vi "Optical Flow Example.vi"() -> ()   [LabVIEW 2011]
uses:
  <vilib>/vision/NI_Vision_Development_Module.lvlib
panel:
  out "Image":T1(plugin-control)
  in  "stop":bool
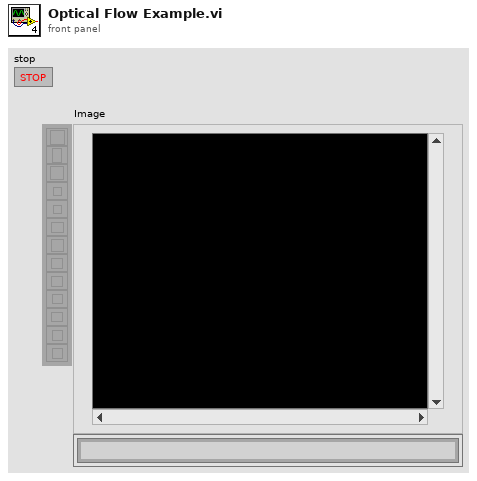
[diagram p1: front panel]
types:
  T1 = typedef "IMAQ Image.ctl" = refnum<image>
  T2 = typedef "Image Type" = u32
  T3 = typedef "t_CallbackReferences.ctl" = cluster{"LV event callback ":refnum<k27>, "Proxy instance":refnum<k24>, "(*f)(...)":i32}
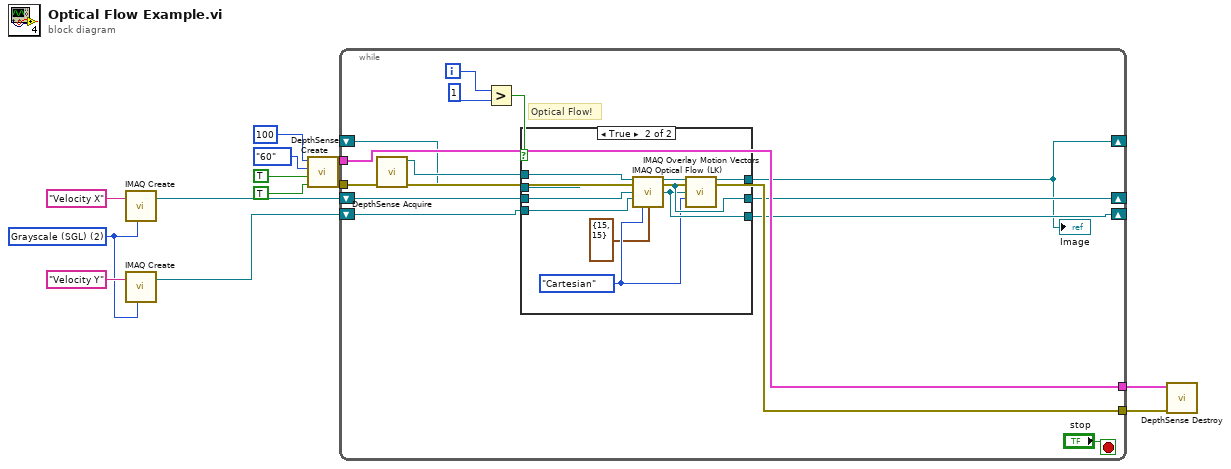
[diagram p0: block diagram]
diagram:
  w3 = T2 2 items=["Grayscale (U8)", "Grayscale (I16)", "Grayscale (SGL)", "Complex (CSG)", "RGB (U32)", "HSL (U32)", "RGB (U64)", "Grayscale (U16)"] ("Image Type")
  n1 = call "IMAQ Create"("Image Name"="Velocity X", "Image Type"=w3) -> ("New Image"=w2:T1)  [unwired: 2 in, 2 out]
  n2 = call "IMAQ Create"("Image Name"="Velocity Y", "Image Type"=w3) -> ("New Image"=w1:T1)  [unwired: 2 in, 2 out]
  n3 = call "DepthSense Create.vi"("Denoise?"=TRUE, "Close Mode?"=TRUE, "Framerate"=enum32{"25", "30", "50", "60"}."60", "Confidence"=100) -> ("error out"=w13:errorcluster, "callbacks"=w11:cluster{"References":T3, "References":T3})  [unwired: 5 in, 1 out]
  n4 = while {
    tunnel: w13 -> [w27]
    tunnel: [w25] -> w12
    tunnel: [w24] -> w10
    tunnel: w11 -> [w24]
    shift-right: [w22] -> _
    shift-left: w1 -> [w18]
    shift-right: [w23] -> _
    shift-left: w2 -> [w19]
    shift-right: [w14] -> _
    shift-left: _ -> [w20]
    i -> [w17]
    stop <- "stop" stop-if-true
    # "Optical Flow!"
    n5 = call "DepthSense Acquire.vi"("error in (no error)"=w27) -> ("error out"=w25:errorcluster, "new depth frame"=w21:T1)  [unwired: 9 in]
    n6 = Greater?(x=w17, y=1) -> (0:w15:bool)
    n7 = case shown="True" w15 {
      tunnel: [w30 w36] -> w23
      tunnel: [w29 w35] -> w22
      tunnel: w21 -> [w28 w40]
      tunnel: w20 -> [_ w39]
      tunnel: w19 -> [w30 w38]
      tunnel: w18 -> [w29 w37]
      tunnel: [w28 w33] -> w14
      frame False {
      }
      frame True {
        w32 = enum16{"Cartesian", "Polar"}."Cartesian" ("Velocity Representation")
        n8 = call "IMAQ Optical Flow (LK)"("Current Frame"=w40, "Previous Frame"=w39, "Velocity Component 1 In"=w38, "Velocity Component 2 In"=w37, "Velocity Representation"=w32, "Window Size (15x15)"=cluster{"SizeX":i32, "SizeY":i32} {"SizeX"=15, "SizeY"=15}) -> ("Current Frame Out (dup)"=w34:T1, "Velocity Component 1 Out"=w36:T1, "Velocity Component 2 Out"=w35:T1)  [unwired: 6 in, 1 out]
        n9 = call "IMAQ Overlay Motion Vectors"("Image"=w34, "Velocity Component 1"=w36, "Velocity Component 2"=w35, "Velocity Representation"=w32) -> ("Image Out"=w33:T1)  [unwired: 10 in, 1 out]
      }
    }
    "Image" <- w14
  }
  n10 = call "DepthSense Destroy.vi"("error in (no error)"=w12, "callbacks"=w10) -> ()  [unwired: 10 in]
